vi "Deconstruct PDU.vi"(8 "error in (no error)":errorcluster, 11 "Modbus data unit in":refnum<class "Modbus Data Unit (PDU).lvclass">) -> (0 "error out":errorcluster, 2 "data":u8[](array[numeric]), 3 "function":u8(ring) items=["Read Discrete Inputs"=2, "Read Coils"=1, "Write Single Coil"=5, "Write Multiple Coils"=15, "Read Input Register"=4, "Read Holding Registers"=3, "Write Single Register"=6, "Write Multiple Registers"=16, "Read/Write Multiple Registers"=23, "Mask Write Register"=22, "Read FIFO Queue"=24, "Read File Record"=20, "Write File Record"=21, "Read Exception Status"=7, "Diagnostic"=8, "Get Com Event Counter"=11, "Get Com Event Log"=12, "Report Slave ID"=17, "Read Device Identification"=43])   [LabVIEW 2020, in "SubVIs.lvlib" / "Modbus Data Unit (PDU).lvclass"]
uses:
  <vilib>/Modbus/subvis/Modbus Data Unit (PDU)/Modbus Data Unit (PDU).lvclass
  <vilib>/Modbus/subvis/Modbus Data Unit (PDU)/Modbus Data Unit (PDU).lvclass/Modbus Data Unit (PDU).ctl
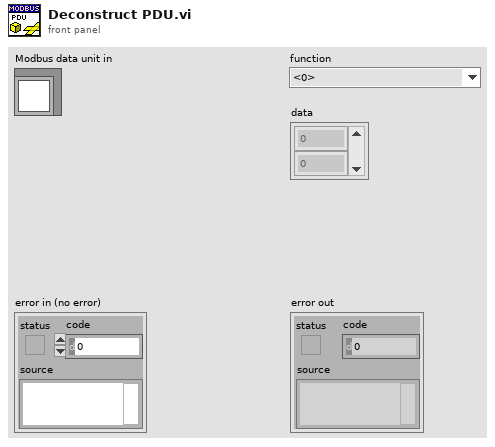
[diagram p1: front panel]
types:
  T1 = typedef "SubVIs.lvlib/Modbus Data Unit (PDU).lvclass/Function.ctl" = u8
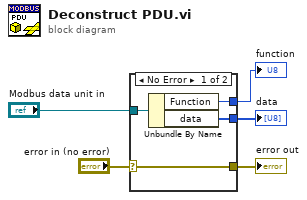
[diagram p0: block diagram]
diagram:
  n1 = case shown="No Error" "error in (no error)" {
    selector: "error in (no error)" -> [w6 w10]
    tunnel: "Modbus data unit in" -> [w9 _]
    tunnel: [w8 _] -> w4
    tunnel: [w7 _] -> w3
    tunnel: [w6 w10] -> w1
    frame No Error {
      n2 = Unbundle By Name(w9) -> ("Function"=w8:T1, "data"=w7:u8[])
    }
    frame Error {
    }
  }
  "error out" <- w1
  "function" <- w4
  "data" <- w3
